vi "Stop Core.vi"(10 "final error code":i32, 11 "Nested in":refnum<class "Mech Pump.lvclass">) -> (3 "Nested out":refnum<class "Mech Pump.lvclass">)   [LabVIEW 2021, in "Mech Pump.lvlib" / "Mech Pump.lvclass"]
doc: "(<B>Filename</B>: Actor Framework.lvlib:Actor.lvclass:Stop Core.vi)\n\nDefines what the actor does before it stops. Use the <B>final error code</B> input to determine whether the actor shut down in response to an error.\n\nBy default, this method does nothing. A descendant class may override it to define behavior, such as shutting down any processes the actor initiated in its override of the Actor Core method."
uses:
  Mech Pump.lvclass
  Mech Pump.lvclass/Mech Pump.ctl
  <vilib>/MGI/Panel Manager/Panel Actor/Panel Actor/Panel Actor.lvclass
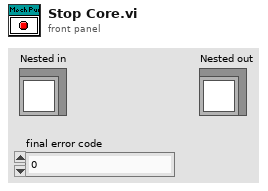
[diagram p1: front panel]
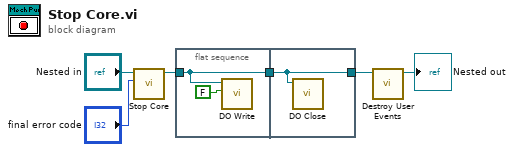
[diagram p0: block diagram]
diagram:
  n1 = call-parent "Stop Core.vi"("final error code"="final error code", "Actor in"="Nested in") -> ("Actor out"=w3:refnum<class "Mech Pump.lvclass">)  [unwired: 9 in]
  n2 = flat-sequence {
    tunnel: w3 -> [w7]
    tunnel: [w7] -> w1
    tunnel: [w9] -> w2
    tunnel: w1 -> [w9]
    frame #0 {
      n3 = call "DO Write.vi"("Digital Output"=FALSE, "Mech Pump in"=w7) -> ()  [unwired: 9 in, 1 out]
    }
    frame #1 {
      n4 = call "DO Close.vi"("Mech Pump in"=w9) -> ()  [unwired: 10 in, 1 out]
    }
  }
  n5 = call "Destroy User Events.vi"("UI Template in"=w2) -> ("UI Template out"=→"Nested out":refnum<class "Mech Pump.lvclass">)  [unwired: 10 in]
